vi "Theta change.vi"(9 "Theta":dbl(knob) scale=0.0..360.0, 11 "Original Graph":T2(graph) caption="cpsgraph") -> (0 "StdDev of Y":sgl, 1 "array of new data":dbl[][](array[numeric]), 3 "Rotated Graph":T1(graph) caption="cpsgraph")   [LabVIEW 2023]
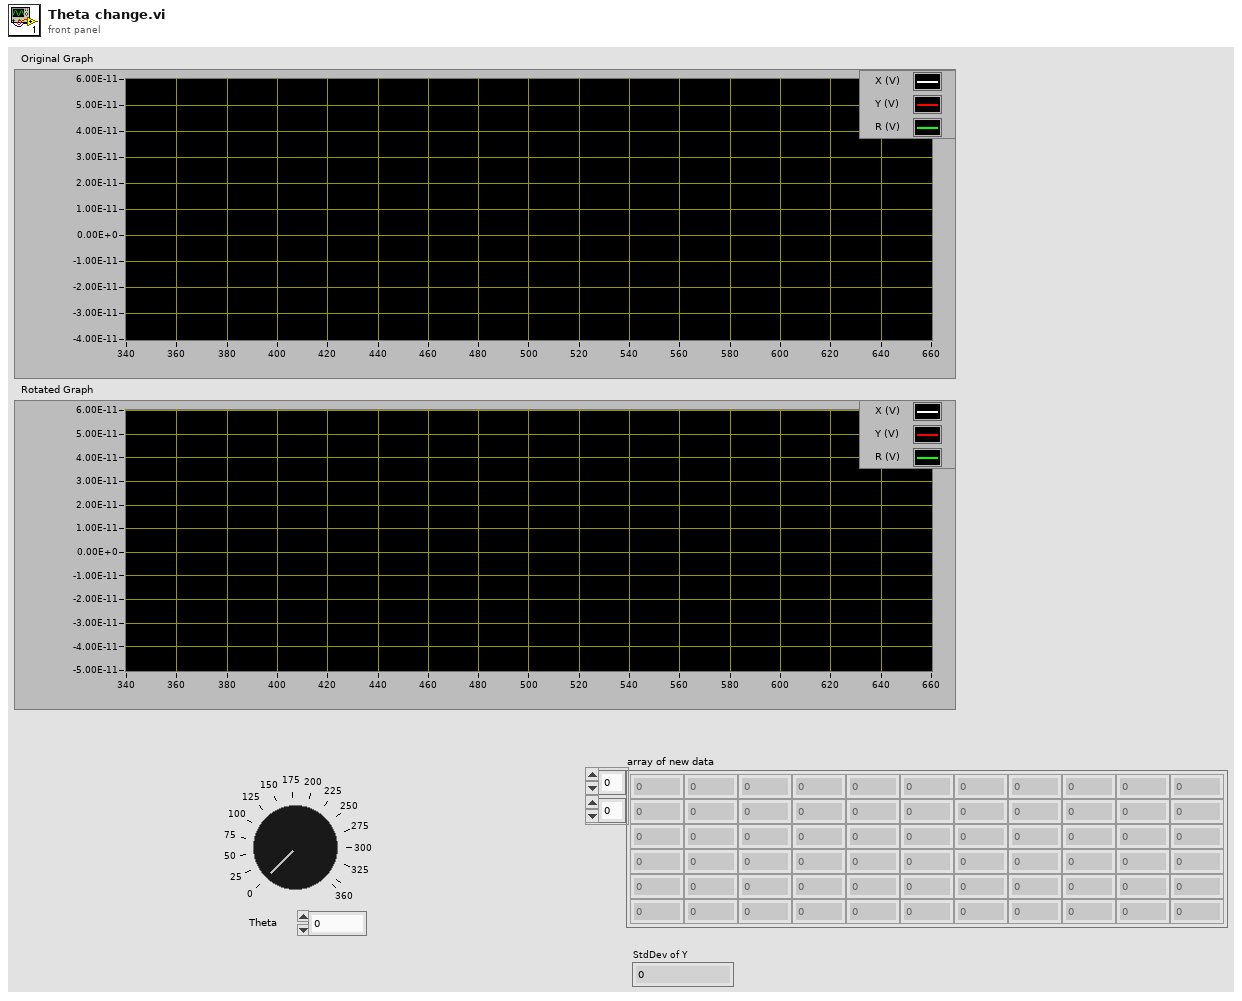
[diagram p1: front panel]
types:
  T1 = cluster{"point array":cluster{"x":dbl, "y":dbl}[]}[]
  T2 = typedef "Scan Driver.lvclass/Scan Graph.ctl" = cluster{"point array":cluster{"x":dbl, "y":dbl}[]}[]
  T3 = cluster{"point array":cluster{"x":dbl, "y":dbl}[]}
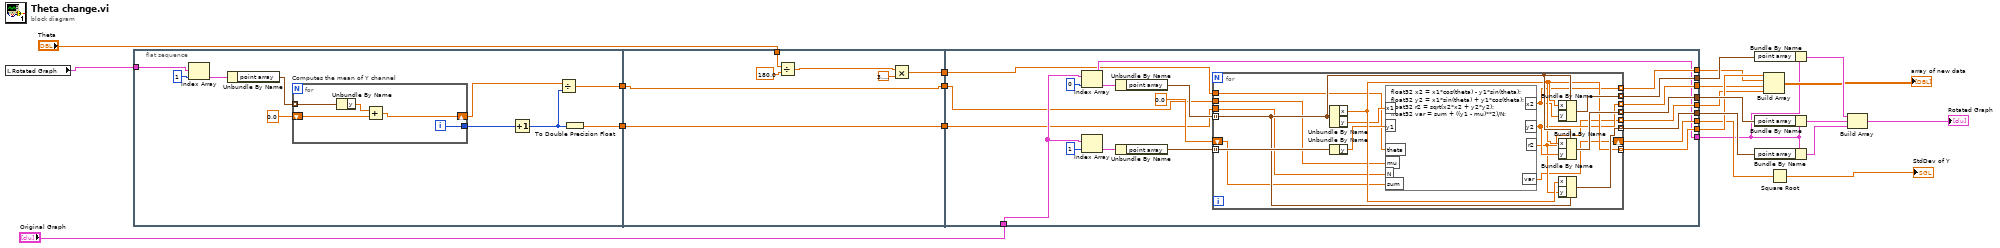
[diagram p0: block diagram]
diagram:
  n1 = local read "Rotated Graph"() -> (w1:T1)
  n2 = flat-sequence {
    tunnel: [w26] -> w23
    tunnel: [w25] -> w22
    tunnel: w1 -> [w24]
    tunnel: w23 -> [w42]
    tunnel: [w43] -> w21
    tunnel: w22 -> [w43]
    tunnel: [w42] -> w20
    tunnel: [w41] -> w19
    tunnel: "Theta" -> [w39]
    tunnel: [w64] -> w15
    tunnel: [w63] -> w14
    tunnel: [w62] -> w13
    tunnel: [w61] -> w12
    tunnel: [w60] -> w11
    tunnel: [w59] -> w10
    tunnel: [w58] -> w9
    tunnel: [w57] -> w7
    tunnel: "Original Graph" -> [w51]
    tunnel: [w50] -> w4
    tunnel: w21 -> [w49]
    tunnel: w20 -> [w48]
    tunnel: w19 -> [w47]
    frame #0 {
      n3 = Index Array(array=w24, index=1) -> (element=w27:T3)
      n4 = Unbundle By Name(w27) -> ("point array"=w28:cluster{"x":dbl, "y":dbl}[])
      n5 = for "Computes the mean of Y channel" {
        tunnel: w28 -> [w35] mode=indexing
        shift-right: [w37] -> w31
        shift-left: 0.0 -> [w38]
        tunnel: [w36] -> w30
        i -> [w36]
        n6 = Unbundle By Name(w35) -> ("y"=w34:dbl)
        n7 = Add(x=w34, y=w38) -> (x+y=w37:dbl)
      }
      n8 = Increment(x=w30) -> (x+1=w32:i32)
      n9 = Divide(x=w31, y=w32) -> (x/y=w26:dbl)
      n10 = To Double Precision Float(number=w32) -> (double precision float=w25:dbl)
    }
    frame #1 {
      n11 = Divide(x=w39, y=180.0) -> (x/y=w44:dbl)
      n12 = Multiply(x=w44, y=3.141592653589793) -> (x*y=w41:dbl)
    }
    frame #2 {
      n13 = Index Array(array=w51, index=0) -> (element=w50:T3)
      n14 = Index Array(array=w51, index=1) -> (element=w54:T3)
      n15 = Unbundle By Name(w50) -> ("point array"=w53:cluster{"x":dbl, "y":dbl}[])
      n16 = Unbundle By Name(w54) -> ("point array"=w52:cluster{"x":dbl, "y":dbl}[])
      n17 = for {
        tunnel: w53 -> [w79] mode=indexing
        tunnel: w52 -> [w80] mode=indexing
        tunnel: w47 -> [w72]
        tunnel: [w78] -> w62 mode=indexing
        tunnel: [w77] -> w63 mode=indexing
        tunnel: [w76] -> w64 mode=indexing
        tunnel: [w75] -> w61 mode=indexing
        tunnel: [w71] -> w60 mode=indexing
        tunnel: [w70] -> w59 mode=indexing
        tunnel: [w69] -> w58 mode=indexing
        shift-right: [w68] -> w57
        shift-left: sgl 0.0 -> [w67]
        tunnel: w49 -> [w66]
        tunnel: w48 -> [w65]
        n18 = Unbundle By Name(w79) -> ("x"=w75:dbl, "y"=w74:dbl)
        n19 = Unbundle By Name(w80) -> ("y"=w73:dbl)
        n20 = formula code="float32 x2 = x1*cos(theta) - y1*sin(theta);\nfloat32 y2 = x1*sin(theta) + y1*cos(theta);\nfloat32 r2 = sqrt(x2*x2 + y2*y2);\nfloat32 var = sum + ((y1 - mu)**2)/N;"("x1"=w74, "y1"=w73, "theta"=w72, "mu"=w65, "N"=w66, "sum"=w67) -> ("x2"=w71:sgl, "y2"=w70:sgl, "r2"=w69:sgl, "var"=w68:sgl)
        n21 = Bundle By Name(cluster=w79, "x"=w75, "y"=w71) -> (w78:cluster{"x":dbl, "y":dbl})
        n22 = Bundle By Name(cluster=w79, "x"=w75, "y"=w70) -> (w77:cluster{"x":dbl, "y":dbl})
        n23 = Bundle By Name(cluster=w79, "x"=w75, "y"=w69) -> (w76:cluster{"x":dbl, "y":dbl})
      }
    }
  }
  n24 = Bundle By Name(cluster=w4, "point array"=w13) -> (w16:T3)
  n25 = Bundle By Name(cluster=w4, "point array"=w14) -> (w17:T3)
  n26 = Bundle By Name(cluster=w4, "point array"=w15) -> (w18:T3)
  n27 = Build Array(w12, w11, w10, w9) -> (→"array of new data":dbl[][])
  n28 = Square Root(x=w7) -> (sqrt(x)=→"StdDev of Y":sgl)
  n29 = Build Array(w16, w17, w18) -> (→"Rotated Graph":T1)
